vi "waveform_to_script.vi"(6 "Hardware alignment quantum (in samples)":u16=1 min=1 step=1, 8 "Data":u32[](array[numeric]) format="%08x", 9 "existing waveform samples (in)":u32[](array[numeric]), 10 "existing waveform names":string[](array[string]), 11 "Transitions (sorted and reduced)":u32[](array[numeric])) -> (0 "script":string, 1 "waveform samples (out)":u32[](array[numeric]), 2 "Some sample was padded?":bool, 3 "waveform names":string[](array[string]))   [LabVIEW 2013]
panel:
  out "Gap":u32[](array[numeric])
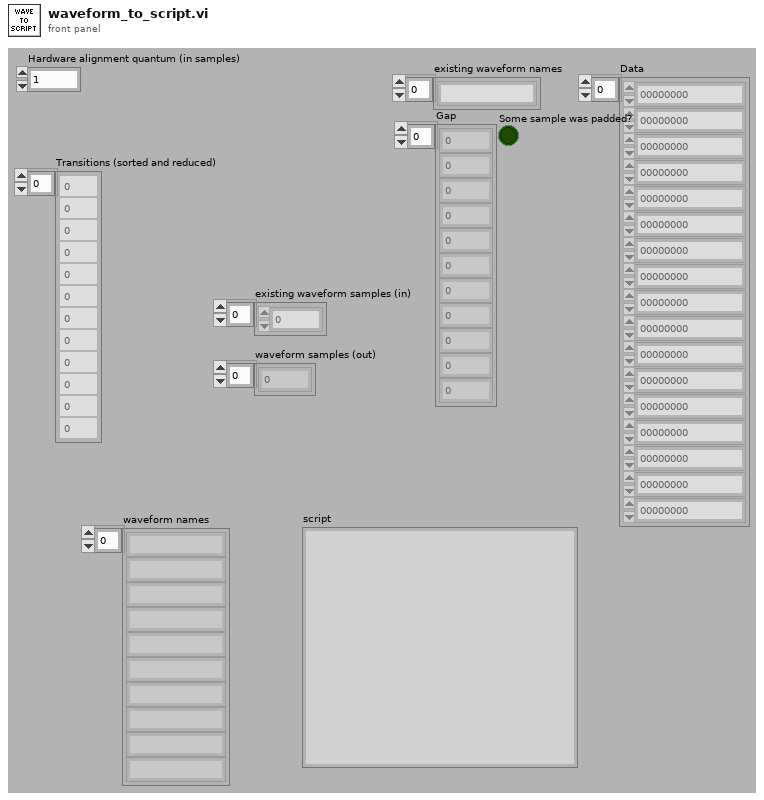
[diagram p1: front panel]
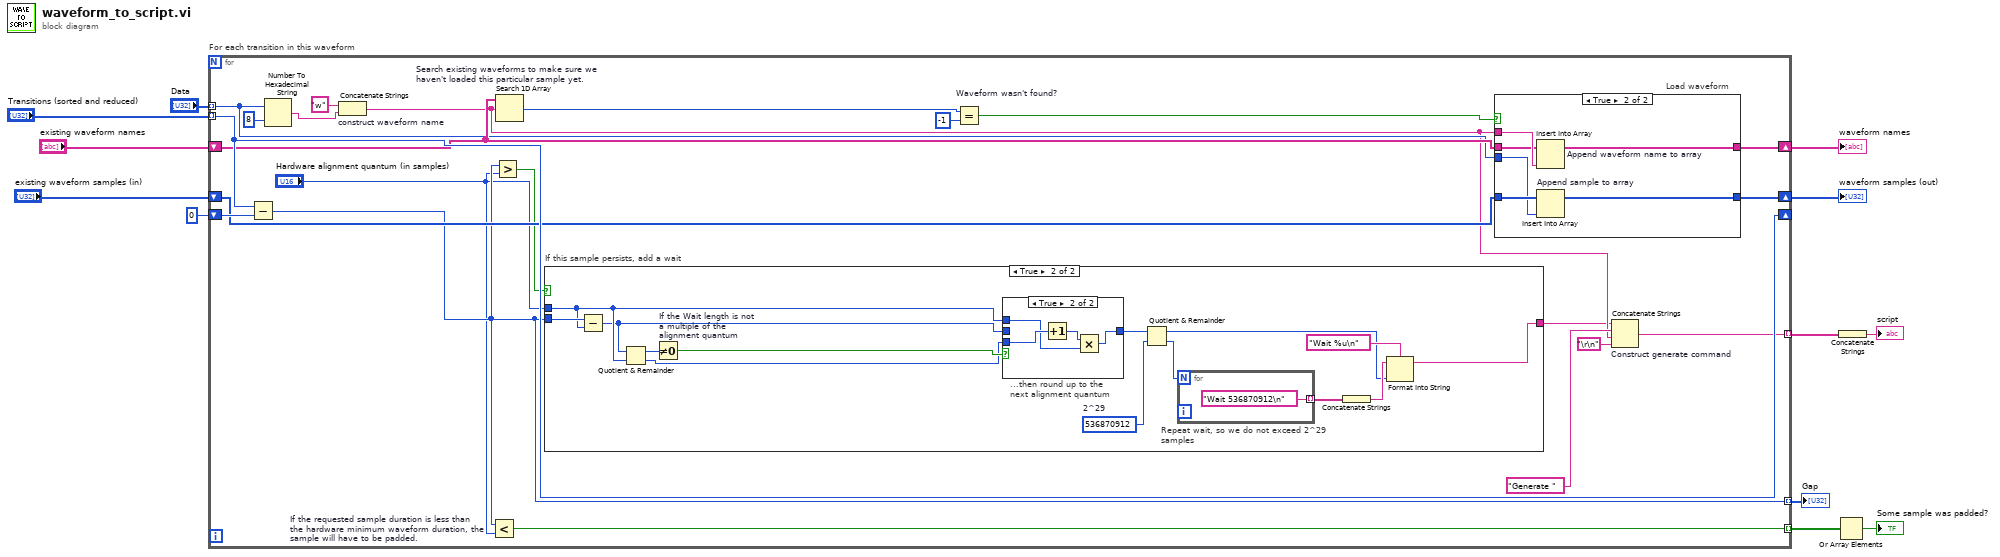
[diagram p0: block diagram]
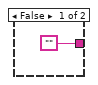
[diagram p3: hidden frame]
diagram:
  n1 = for "For each transition in this waveform" {
    tunnel: "Transitions (sorted and reduced)" -> [w34] mode=indexing
    shift-right: [w34] -> _
    shift-left: u32 0 -> [w33]
    shift-right: [w23] -> w7
    shift-left: "existing waveform names" -> [w24]
    tunnel: "Data" -> [w21] mode=indexing
    shift-right: [w20] -> w3
    shift-left: "existing waveform samples (in)" -> [w22]
    tunnel: [w17] -> w6 mode=indexing
    tunnel: [w15] -> w4 mode=indexing
    tunnel: [w13] -> w2 mode=indexing
    n2 = Subtract(x=w34, y=w33) -> (x-y=w15:u32)
    n3 = Number To Hexadecimal String(1:i16 8 ("width (-)"), 2:w21) -> (0:w25:string)
    n4 = Concatenate Strings "construct waveform name"("w" ("string"), w25) -> (w19:string)
    n5 = Less? "If the requested sample duration is less than the hardware minimum waveform duration, the sample will have to be padded."(x=w15, y="Hardware alignment quantum (in samples)") -> (x < y?=w13:bool)
    n6 = Greater?(x=w15, y="Hardware alignment quantum (in samples)") -> (0:w16:bool)
    n7 = Search 1D Array "Search existing waveforms to make sure we haven't loaded this particular sample yet."(1D array=w24, element=w19) -> (index of element=w29:i32)  [unwired: 1 in]
    n8 = case "If this sample persists, add a wait" shown="True" w16 {
      tunnel: w15 -> [_ w50]
      tunnel: ["" w56] -> w18
      tunnel: "Hardware alignment quantum (in samples)" -> [_ w45]
      frame False {
      }
      frame True {
        w55 = u32 536870912  # 2^29
        n9 = Subtract(x=w50, y=w45) -> (x-y=w44:u32)
        n10 = Quotient & Remainder(x=w44, y=w45) -> (x-y*floor(x/y)=w49:u32, floor(x/y)=w46:u32)
        n11 = Not Equal To 0? "If the Wait length is not a multiple of the alignment quantum"(x=w49) -> (x != 0?=w48:bool)
        n12 = case "...then round up to the next alignment quantum" shown="True" w48 {
          tunnel: [w58 w59] -> w47
          tunnel: w46 -> [_ w62]
          tunnel: w45 -> [_ w60]
          tunnel: w44 -> [w58 _]
          frame False {
          }
          frame True {
            n13 = Increment(x=w62) -> (x+1=w61:u32)
            n14 = Multiply(x=w61, y=w60) -> (x*y=w59:u32)
          }
        }
        n15 = Quotient & Remainder(x=w47, y=w55) -> (x-y*floor(x/y)=w51:u32, floor(x/y)=w54:u32)
        n16 = for "Repeat wait, so we do not exceed 2^29 samples" {
          N: w54 -> [_]
          tunnel: ["Wait 536870912\n" ("format string")] -> w53 mode=indexing
        }
        n17 = Concatenate Strings(w53) -> (w52:string)
        n18 = Format Into String "Format Into String"(format string="Wait %u\n", initial string=w52, w51) -> (resulting string=w56:string)  [unwired: 1 in, 1 out]
      }
    }
    n19 = Equal? "Waveform wasn't found?"(x=w29, y=-1) -> (x = y?=w30:bool)
    n20 = case "Load waveform" shown="True" w30 {
      tunnel: w19 -> [_ w42]
      tunnel: w24 -> [w36 w41]
      tunnel: [w36 w40] -> w23
      tunnel: w22 -> [w35 w39]
      tunnel: w21 -> [_ w38]
      tunnel: [w35 w37] -> w20
      frame False {
      }
      frame True {
        n21 = Insert Into Array "Append waveform name to array"(array=w41, new element=w42) -> (w40:string[])  [unwired: 1 in]
        n22 = Insert Into Array "Append sample to array"(array=w39, new element=w38) -> (w37:u32[])  [unwired: 1 in]
      }
    }
    n23 = Concatenate Strings "Construct generate command"(w18, "Generate ", w19, "\r\n") -> (w17:string)
  }
  "waveform names" <- w7
  "Gap" <- w4
  "waveform samples (out)" <- w3
  n24 = Or Array Elements(Boolean array=w2) -> (logical OR=→"Some sample was padded?":bool)
  n25 = Concatenate Strings(w6) -> (→"script":string)
